vi "Callback..FGV.vi"(8 "error in (no error)":errorcluster) -> (0 "error out":errorcluster, 3 "Events":T1)   [LabVIEW 2019, in "LabSFTP.lvlib"]
uses:
  LabSFTP.lvlib
  Event Refs.ctl
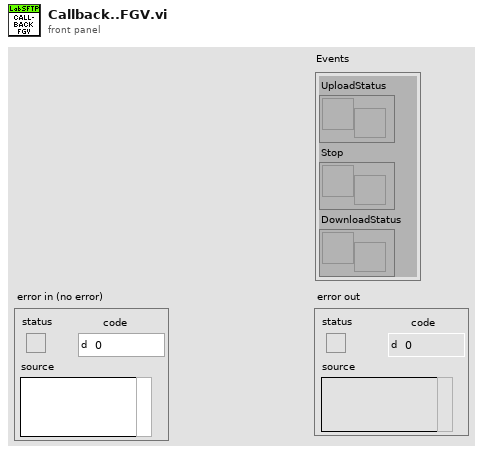
[diagram p1: front panel]
types:
  T1 = typedef "LabSFTP.lvlib/Event Refs.ctl" = cluster{"UploadStatus":refnum<user-event>, "Stop":refnum<user-event>, "DownloadStatus":refnum<user-event>}
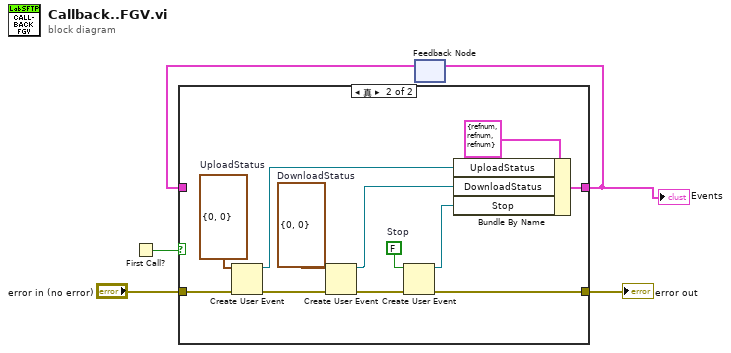
[diagram p0: block diagram]
diagram:
  n1 = First Call?() -> (First Call?: T/F=w2:bool)
  n2 = feedback #1() -> (w3:T1)  [unwired: 1 in]
  n3 = case shown="真" w2 {
    tunnel: "error in (no error)" -> [w6 w18]
    tunnel: [w6 w16] -> w4
    tunnel: [w7 w14] -> w1
    tunnel: w3 -> [w7 _]
    frame False {
    }
    frame True {
      w11 = cluster{"fileSize":i64, "status":u64} {"fileSize"=0, "status"=0}  # DownloadStatus
      w15 = FALSE  # Stop
      w19 = cluster{"fileSize":i64, "status":u64} {"fileSize"=0, "status"=0}  # UploadStatus
      n4 = Create User Event(user event datatype=w19, error in=w18) -> (user event=w13:refnum<user-event>, error out=w10:errorcluster)
      n5 = Create User Event(user event datatype=w11, error in=w10) -> (user event=w8:refnum<user-event>, error out=w9:errorcluster)
      n6 = Create User Event(user event datatype=w15, error in=w9) -> (user event=w12:refnum<user-event>, error out=w16:errorcluster)
      n7 = Bundle By Name(cluster=T1 {"UploadStatus"=refnum, "Stop"=refnum, "DownloadStatus"=refnum} ("Events"), "UploadStatus"=w13, "DownloadStatus"=w8, "Stop"=w12) -> (w14:T1)
    }
  }
  "error out" <- w4
  "Events" <- w1
  n8 = feedback-in #1(w1) -> ()
